vi "Navigate.vi"(0 "reference in":refnum<class "DP_WebView.lvclass">, 1 "URL":string(combo), 3 "Timeout(10000ms)":i32=10000, 5 "Error In":errorcluster) -> (14 "reference out":refnum<class "DP_WebView.lvclass">, 15 "Loaded":bool, 19 "Error Out":errorcluster)   [LabVIEW 2020, in "DP_WebView.lvclass"]
uses:
  DP_WebView.lvclass
  C:/Projects/DependencyViewer/DependencyViewer/DP_WebView_class/data/Microsoft.Web.WebView2.Core.dll
  data/Microsoft.Web.WebView2.Core.dll
  CallBackVIs/Callback_NavigationComplete.vi
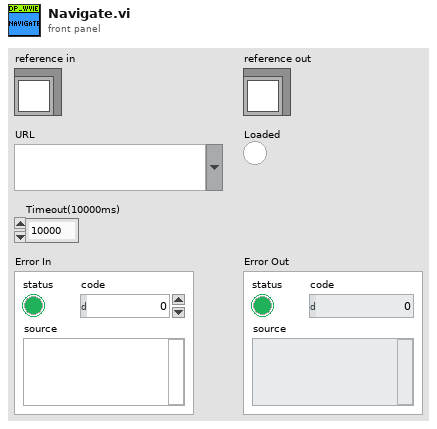
[diagram p1: front panel]
types:
  T1 = typedef "DP_WebView.lvclass/ObjectAttributes.ctl" = cluster{"WebView Container":refnum<k24>, "CoreWebViewRef":refnum<k24>, "Status":i32, "Status Message":string, "User Data Folder":path, "BrowserProcessId":u32}
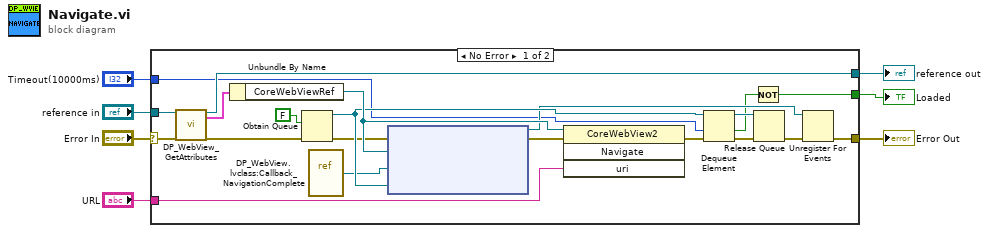
[diagram p0: block diagram]
diagram:
  n1 = case shown="No Error" "Error In" {
    selector: "Error In" -> [w28 w30]
    tunnel: [w22 w30] -> w6
    tunnel: [w26 w29] -> w4
    tunnel: "reference in" -> [w27 w29]
    tunnel: "URL" -> [w24 _]
    tunnel: [w21 _] -> w2
    tunnel: "Timeout(10000ms)" -> [w14 _]
    frame No Error {
      n2 = call "DP_WebView_GetAttributes.vi"("reference in"=w27, "error in (no error)"=w28) -> ("reference out"=w26:refnum<class "DP_WebView.lvclass">, "Data"=w25:T1, "error out"=w17:errorcluster)  [unwired: 14 in, 1 out]
      n3 = Unbundle By Name(w25) -> ("CoreWebViewRef"=w19:refnum<k24>)
      n4 = Obtain Queue(element data type=FALSE ("IsSuccess"), error in (no error)=w17) -> (queue out=w18:refnum<queue>, error out=w16:errorcluster)  [unwired: 3 in, 1 out]
      n5 = vi-ref "DP_WebView.lvclass:Callback_NavigationComplete.vi"() -> ("vi reference"=w13:refnum<vi>)
      n6 = node(w16, w19, w13, w18) -> (w15:refnum<k27>, w20:errorcluster)  [unwired: 1 in]
      n7 = invoke class="CoreWebView2" method="Navigate"(reference=w19, error in=w20, "uri"=w24) -> (error out=w23:errorcluster)  [unwired: 1 in, 3 out]
      n8 = Dequeue Element(queue=w18, timeout in ms (-1)=w14, error in (no error)=w23) -> (queue out=w11:refnum<queue>, timed out?=w8:bool, error out=w10:errorcluster)  [unwired: 1 out]
      n9 = Not(x=w8) -> (.not. x?=w21:bool)
      n10 = Release Queue(queue=w11, error in (no error)=w10) -> (error out=w9:errorcluster)  [unwired: 1 in, 2 out]
      n11 = Unregister For Events(event registration refnum=w15, error in=w9) -> (error out=w22:errorcluster)
    }
    frame Error {
    }
  }
  "Error Out" <- w6
  "reference out" <- w4
  "Loaded" <- w2
